vi "MainNR.vi"(10 "JQMHStartup":refnum<class "RQMHStartup.lvclass">, 11 "NewTemplate in":refnum<class "NewTemplate.lvclass">) -> ()   [LabVIEW 2024, in "NewTemplate.lvclass"]
uses:
  NewTemplate.lvclass
  C:/Github/JQMH/JQMHCore/Module/RQMHModule.lvclass
  JQMHCore/JQMHStartup/RQMHStartup.lvclass
  Message Queue_class/RQMHMessageQueue.lvclass/RQMHMessageQueue.ctl
  JQMHCore/Module/InitialiseReplyArgs.ctl
  <vilib>/Utility/miscctls.llb/LVPointTypeDef.ctl
  JQMHCore/Module/RQMHModule.lvclass/RQMHModule.ctl
  Do Something ReplyArgs.ctl
  Do Something Args.ctl
  JQMHCore/Module/Read ModuleName.vi
  JQMHCore/Module/Read External Start.vi
  Message Queue_class/Delacor_lib_QMH_Enqueue Message (Single).vi
  Message Queue_class/RQMHMessageQueue.lvclass
  JQMHCore/Module/RQMHModule.lvclass
  JQMHCore/Shared/RQMHShared.lvlib
panel:
  out "error out":errorcluster
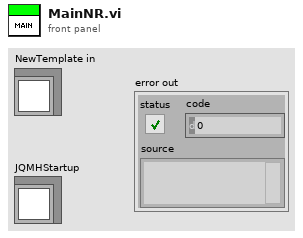
[diagram p1: front panel]
types:
  T1 = typedef "NewTemplate.lvclass/Request Events--cluster.ctl" = cluster{"Do Something":refnum<user-event>}
  T2 = cluster{"Stop Module":refnum<user-event>, "Requests":T1}
  T3 = typedef "LVPointTypeDef.ctl" = cluster{"Horizontal":i16, "Vertical":i16}
  T4 = enum32{"Invalid", "Standard", "Closed", "Hidden", "Minimized", "Maximized"}
  T5 = typedef "RQMHModule.lvclass/InitialiseReplyArgs.ctl" = cluster{"Did Init?":bool}
  T6 = typedef "NewTemplate.lvclass/Do Something Args.ctl" = cluster{"Msg":string}
  T7 = typedef "NewTemplate.lvclass/Do Something ReplyArgs.ctl" = cluster{"Value":dbl, "Boolean":bool}
  T8 = typedef "RQMHModule.lvclass/Reply.ctl" = cluster{"Expects Reply":bool, "Reply":refnum<notifier>}
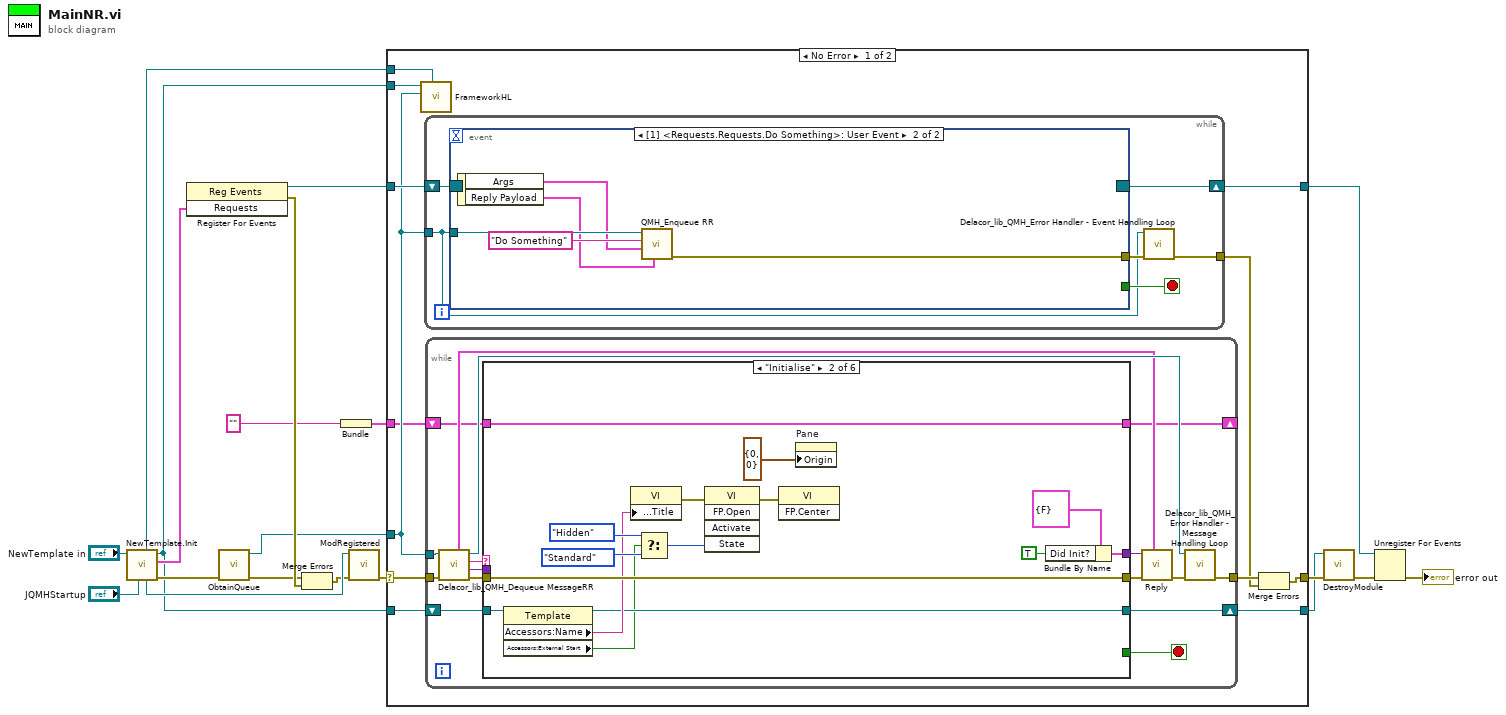
[diagram p0: block diagram]
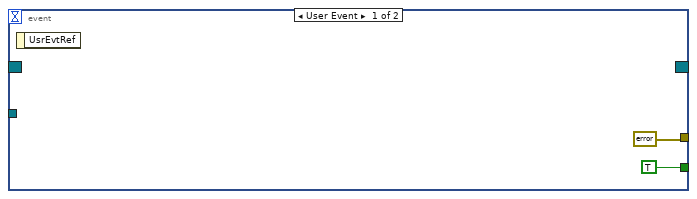
[diagram p2: hidden frame]
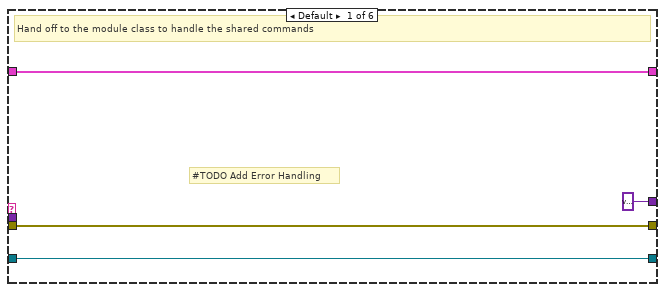
[diagram p3: hidden frame]
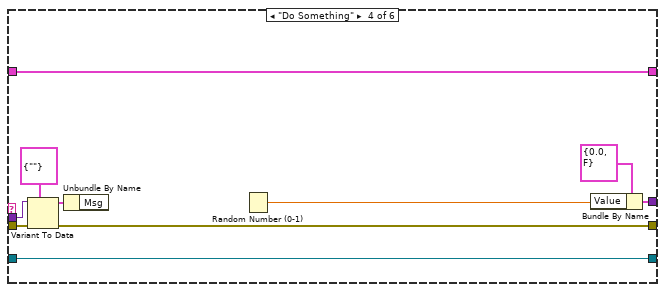
[diagram p5: hidden frame]
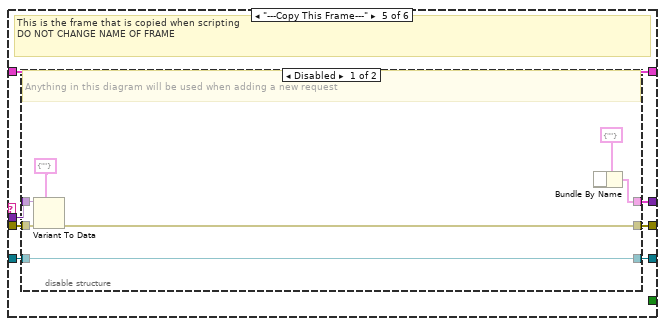
[diagram p6: hidden frame]
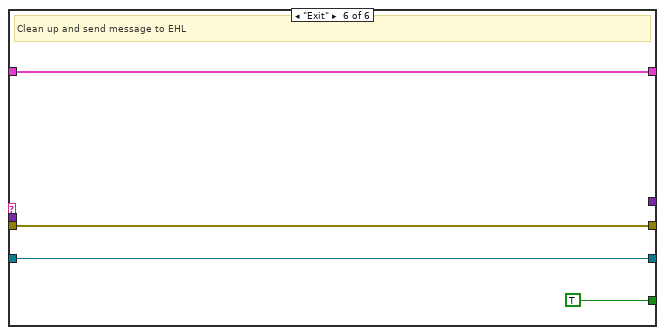
[diagram p8: hidden frame]
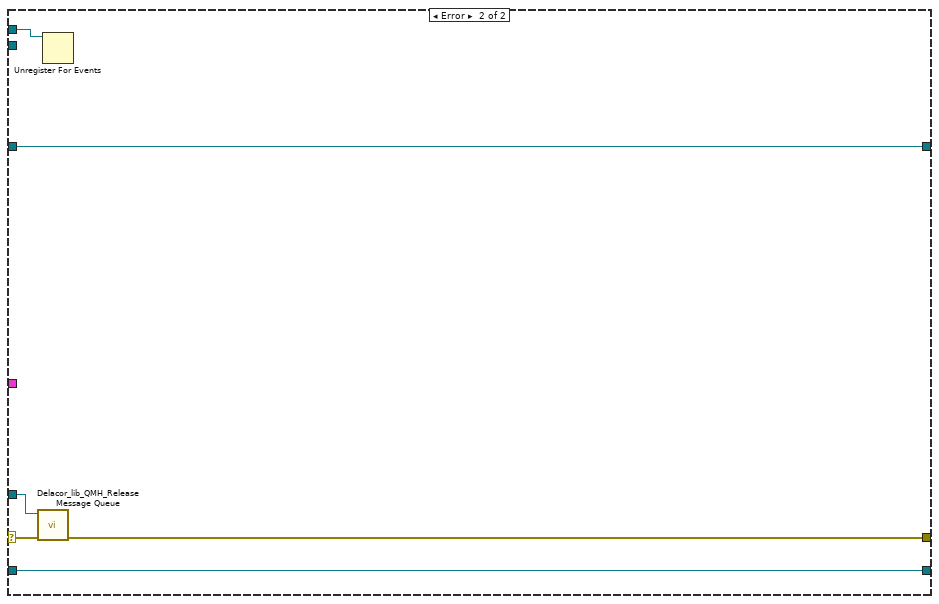
[diagram p9: hidden frame]
diagram:
  n1 = call "NewTemplate.Init.vi"("JQMHStartup in"="JQMHStartup", "NewTemplate in"="NewTemplate in") -> ("error out"=w13:errorcluster, "Requests"=w4:T2, "NewTemplate out"=w3:refnum<class "NewTemplate.lvclass">, "JQMHStartup out"=w11:refnum<class "RQMHStartup.lvclass">, "StandardRequests"=w7:refnum<event-registration>)  [unwired: 3 in, 2 out]
  n2 = register-events(w4) -> (reference out=w6:refnum<event-registration>, error out=w20:errorcluster)  [unwired: 2 in]
  n3 = call "ObtainQueue.vi"("error in"=w13) -> ("error out"=w12:errorcluster, "Message Queue"=w8:refnum<class "RQMHMessageQueue.lvclass">)  [unwired: 9 in]
  n4 = Merge Errors(w12, w20) -> (w9:errorcluster)
  n5 = Bundle("") -> (w2:cluster{string})  [unwired: 1 in]
  n6 = call "ModRegistered.vi"("error in (no error)"=w9, "JQMHStartup in"=w11) -> ("error out"=w10:errorcluster)  [unwired: 9 in]
  n7 = case "RQMH_MAIN" shown="No Error" w10 {
    selector: w10 -> [w29 w117]
    tunnel: w3 -> [w32 w116]
    tunnel: [w31 w119] -> w19
    tunnel: w6 -> [w30 w119]
    tunnel: w8 -> [w23 w118]
    tunnel: [w28 w116] -> w5
    tunnel: [w25 w115] -> w16
    tunnel: w3 -> [w24 _]
    tunnel: w7 -> [w22 w114]
    tunnel: w2 -> [w21 _]
    frame No Error {
      n8 = call-dynamic "FrameworkHL.vi"("StandardRequests"=w22, "Message Queue"=w23, "JQMHModule in"=w24) -> ()  [unwired: 9 in]
      n9 = while {
        shift-right: [w38] -> w31
        shift-left: w30 -> [w33]
        tunnel: w23 -> [w34]
        tunnel: [w35] -> w26
        stop <- w37 stop-if-true
        n10 = event "RQMH_EVENT_MAIN" shown="[1] <Requests.Requests.Do Something>: User Event" {
          selector: w33 -> [_ _]
          dyn-events: [_ _] -> w38
          timeout: _ -> [_ _]
          tunnel: [TRUE _] -> w37
          tunnel: w34 -> [_ w45]
          tunnel: [errorcluster {"status"=FALSE, "code"=0, "source"=""} ("error out") w42] -> w36
          event User Event {
            n11 = event-data() -> ()  [unwired: 1 in, 1 out]
          }
          event User Event {
            n12 = event-data() -> ("Args"=w43:T6, "Reply Payload"=w41:T8)  [unwired: 1 in]
            n13 = call "QMH_Enqueue RR.vi"("Reply"=w41, "Message Data"=w43, "Message"="Do Something", "Message Queue in"=w45) -> ("error out"=w42:errorcluster)  [unwired: 6 in, 1 out]
          }
        }
        n14 = call-dynamic "Delacor_lib_QMH_Error Handler - Event Handling Loop.vi"("error in"=w36, "Message Queue in"=w34) -> ("dup error in"=w35:errorcluster)  [unwired: 8 in, 1 out]
      }
      n15 = while {
        tunnel: w23 -> [w56]
        tunnel: w29 -> [w55]
        shift-right: [w58] -> w28
        shift-left: w32 -> [w59]
        tunnel: [w57] -> w27
        shift-right: [w46] -> _
        shift-left: w21 -> [w47]
        stop <- w61 stop-if-true
        n16 = call-dynamic "Delacor_lib_QMH_Dequeue MessageRR.vi"("error in"=w55, "Message Queue in"=w56) -> ("error out"=w54:errorcluster, "Message Data"=w52:variant, "Message"=w53:string, "Message Queue out"=w60:refnum<class "RQMHMessageQueue.lvclass">, "Reply"=w48:T8)  [unwired: 5 in]
        n17 = case "RQMH_MESSAGE_CASES" shown="\"Initialise\"" w53 {
          tunnel: [_ _ _ _ _ TRUE] -> w61
          tunnel: w59 -> [w64 w68 w82 w93 w98 w112]
          tunnel: w52 -> [_ _ _ w89 w96 _]
          tunnel: w54 -> [w65 w80 w83 w88 w100 w111]
          tunnel: [w65 w80 w83 w87 w99 w111] -> w51
          tunnel: [w64 w69 w82 w93 w97 w112] -> w58
          tunnel: [variant w79 _ w92 w95 _] -> w49
          tunnel: w47 -> [w62 w66 w81 w84 w94 w110]
          tunnel: [w62 w66 w81 w84 w94 w110] -> w46
          frame Default {
            # "#TODO Add Error Handling"
            # "Hand off to the module class to handle the shared commands"
          }
          frame "Initialise" {
            n18 = property class="Template"(reference=w68) -> (reference out=w69:refnum<class "NewTemplate.lvclass">, "Accessors:Name"=w70:string, "Accessors:External Start"=w67:bool)  [unwired: 1 in, 1 out]
            n19 = property on="Property Node" class="VI"("Front Panel.Title"=w70) -> (error out=w77:errorcluster)  [unwired: 2 in, 1 out]
            n20 = Select(t=T4."Hidden" ("State"), s=w67, f=T4."Standard" ("State")) -> (s? t:f=w73:T4)
            n21 = invoke on="Invoke Node" class="VI" method="FP.Open"(error in=w77, "State"=w73) -> (error out=w76:errorcluster)  [unwired: 3 in, 4 out]
            n22 = invoke on="Invoke Node" class="VI" method="FP.Center"(error in=w76) -> ()  [unwired: 2 in, 3 out]
            n23 = property on="Pane" class="Pane"("Origin"=T3 {"Horizontal"=0, "Vertical"=0}) -> ()  [unwired: 2 in, 2 out]
            n24 = Bundle By Name(cluster=T5 {"Did Init?"=FALSE} ("Args"), "Did Init?"=TRUE) -> (w79:T5)
          }
          frame "---Module Specific---" {
          }
          frame "Do Something" {
            n25 = Variant To Data(error in=w88, type=T6 {"Msg"=""} ("Do Something Args"), Variant=w89) -> (data=w85:T6, error out=w87:errorcluster)
            n26 = Unbundle By Name(w85) -> ()  [unwired: 1 out]
            n27 = Random Number (0-1)() -> (number: 0 to 1=w90:dbl)
            n28 = Bundle By Name(cluster=T7 {"Value"=0.0, "Boolean"=FALSE}, "Value"=w90) -> (w92:T7)
          }
          frame "---Copy This Frame---" {
            # "This is the frame that is copied when scripting\nDO NOT CHANGE NAME OF FRAME"
            n29 = disable-structure shown="Disabled" {
              disable-tunnel: w100 -> [w104 w109]
              disable-tunnel: [w105 w109] -> w99
              disable-tunnel: w98 -> [w107 w108]
              disable-tunnel: [w107 w108] -> w97
              disable-tunnel: w96 -> [w106 _]
              disable-tunnel: [w102 _] -> w95
              frame Disabled {
                # "Anything in this diagram will be used when adding a new request"
                n30 = Variant To Data(error in=w104, type=cluster{string} {""} ("RQMH_MHL_MSG_PL"), Variant=w106) -> (error out=w105:errorcluster)  [unwired: 1 out]
                n31 = Bundle By Name(cluster=cluster{string} {""} ("RQMH_MHL_REPLY_PL")) -> (w102:cluster{string})  [unwired: 1 in]
              }
              frame Enabled {
              }
            }
          }
          frame "Exit" {
            # "Clean up and send message to EHL"
          }
        }
        n32 = call "Reply.vi"("Reply"=w48, "error in (no error)"=w51, "ReplyPayload"=w49) -> ("error out"=w50:errorcluster)  [unwired: 8 in]
        n33 = call-dynamic "Delacor_lib_QMH_Error Handler - Message Handling Loop.vi"("error in"=w50, "Message Queue in"=w60) -> ("dup error in"=w57:errorcluster)  [unwired: 8 in, 1 out]
      }
      n34 = Merge Errors(w27, w26) -> (w25:errorcluster)
    }
    frame Error {
      n35 = call-dynamic "Delacor_lib_QMH_Release Message Queue.vi"("error in"=w117, "Message Queue"=w118) -> ("error out"=w115:errorcluster)  [unwired: 9 in]
      n36 = Unregister For Events(event registration refnum=w114) -> ()  [unwired: 1 in, 1 out]
    }
  }
  n37 = call "DestroyModule.vi"("error in (no error)"=w16, "JQMHModule in"=w5) -> ("error out"=w18:errorcluster)  [unwired: 9 in]
  n38 = Unregister For Events(event registration refnum=w19, error in=w18) -> (error out=→"error out":errorcluster)
